vi "create incident - error.vi"(8 "error":errorcluster, 11 "RT Queues":T1) -> (3 "RT Queues out":T1)   [LabVIEW 2018]
uses:
  Type Defs/Queues cluster.ctl
  ICL-LabVIEW_General/Message Scheduler/message scheduler.lvclass
  Type Defs/error incident cluster.ctl
  Queue VIs/En-queue RT comms element.vi
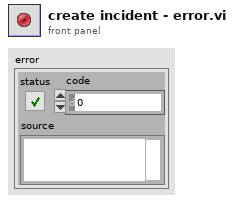
[diagram p1: front panel]
types:
  T1 = typedef "Queues cluster.ctl" = cluster{"RT Message":refnum<queue>, "RT Comms":refnum<queue>, "RT Data":refnum<queue>, "RT FIFO":refnum<queue>, "message scheduler":refnum<class "message scheduler.lvclass">}
  T2 = typedef "error incident cluster.ctl" = cluster{"description":string, "call chain":string[], "error":errorcluster}
  T3 = cluster{"seconds since 1Jan1904":timestamp, "type":string, "Variant":variant}
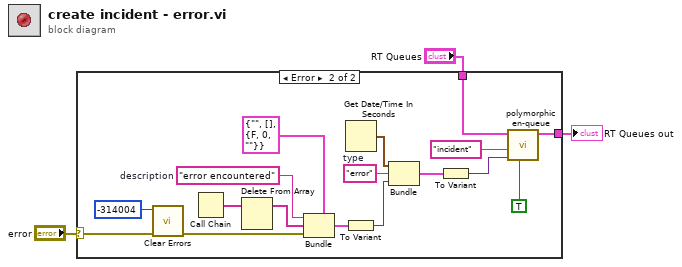
[diagram p0: block diagram]
diagram:
  n1 = case shown="Error" "error" {
    selector: "error" -> [_ w11]
    tunnel: [w4 w7] -> w1
    tunnel: "RT Queues" -> [w4 w6]
    frame No Error {
    }
    frame Error {
      w19 = "error"  # type
      w13 = "error encountered"  # description
      n2 = call <vilib>:"Clear Errors.vi"("error in (no error)"=w11, "specific error code to clear (0: all)"=-314004) -> ("error out"=w10:errorcluster)  [unwired: 4 in, 1 out]
      n3 = Call Chain() -> (call chain=w21:string[])
      n4 = Delete From Array(array=w21) -> (array with subset deleted=w8:string[])  [unwired: 2 in, 1 out]
      n5 = Bundle(cluster=T2 {"description"="", "call chain"=[], "error"={"status"=FALSE, "code"=0, "source"=""}}, "description"=w13, "call chain"=w8, "error"=w10) -> (w18:T2)
      n6 = Get Date/Time In Seconds() -> (seconds since 1Jan1904=w14:timestamp)
      n7 = To Variant(anything=w18) -> (Variant=w17:variant)
      n8 = Bundle("seconds since 1Jan1904"=w14, "type"=w19, "Variant"=w17) -> (w16:T3)  [unwired: 1 in]
      n9 = To Variant(anything=w16) -> (Variant=w15:variant)
      n10 = call-poly "polymorphic en-queue.vi"("prioritise (F)"=TRUE, "Data"=w15, "Message"="incident", "RT Queues"=w6) -> ("RT Queues out"=w7:T1)  [unwired: 7 in]
    }
  }
  "RT Queues out" <- w1
